vi "查询数据.vi"(5 "condition":string, 7 "columns":string[](array[string]), 8 "error in (no error)":errorcluster, 10 "database":string, 11 "table":string) -> (0 "error out":errorcluster, 3 "data":variant[][](array[variant]))   [LabVIEW 2016, in "斯坦道氨氮.lvlib"]
uses:
  <vilib>/Utility/sysdir.llb/System Directory Type.ctl
  <vilib>/addons/database/Connection.llb/DB Tools Open Connec (String).vi
  <vilib>/addons/database/NI_Database_API.lvlib
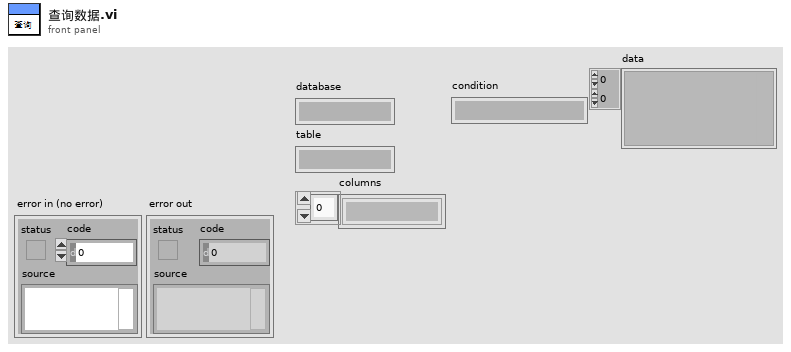
[diagram p1: front panel]
types:
  T1 = typedef "System Directory Type.ctl" = i32
  T2 = typedef "NI_Database_API.lvlib/Conn ObjectReference.ctl" = refnum<k1>
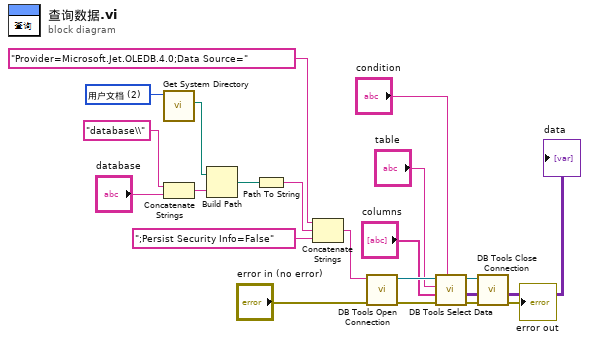
[diagram p0: block diagram]
diagram:
  w12 = T1 2 items=["用户目录"=0, "用户桌面"=1, "用户文档"=2, "用户应用程序数据"=3, "用户设置"=4, "用户临时目录"=5, "公共文档"=6, "公共应用程序数据"=7, "公共设置"=8, "公共缓存"=13, "系统核心库"=9, "系统安装库"=10, "应用程序文件"=11, "启动盘根目录"=12] ("system directory type")
  n1 = call <vilib>:"Get System Directory.vi"("system directory type"=w12) -> ("system directory"=w10:path)  [unwired: 10 in]
  n2 = Concatenate Strings("database\\" ("condition"), "database") -> (w4:string)
  n3 = Build Path(base path=w10, name or relative path=w4) -> (appended path=w9:path)
  n4 = Path To String(path=w9) -> (string=w8:string)
  n5 = Concatenate Strings("Provider=Microsoft.Jet.OLEDB.4.0;Data Source=" ("condition"), w8, ";Persist Security Info=False" ("condition")) -> (w6:string)
  n6 = call-poly <vilib>:"DB Tools Open Connection.vi"("error in (no error)"="error in (no error)", "connection information"=w6) -> ("error out"=w18:errorcluster, "connection reference"=w20:T2)  [unwired: 6 in]
  n7 = call <vilib>:"DB Tools Select Data.vi"("condition"="condition", "error in (no error)"=w18, "columns"="columns", "table"="table", "connection reference"=w20) -> ("error out"=w17:errorcluster, "data"=→"data":variant[][], "connection reference out"=w19:T2)  [unwired: 1 in]
  n8 = call <vilib>:"DB Tools Close Connection.vi"("error in (no error)"=w17, "connection reference"=w19) -> ("error out"=→"error out":errorcluster)  [unwired: 5 in]
